vi "Parse DB - 1553 - Get BM Config.vi"(0 "channel config handle":u32, 11 "error in (no error)":errorcluster) -> (4 "channel config handle out":u32, 6 "Bus_Monitor":T1, 8 "Address Set Inverted":bool, 15 "error out":errorcluster)   [LabVIEW 2013]
uses:
  Controls/1553_Bus_Monitor.ctl
  Controls/1553_BM_Message.ctl
  Controls/664 -Param.ctl
  Controls/1553_Bus_Controller.ctl
  Controls/1553_BC_Message.ctl
  Controls/1553_Acyclic_Frame.ctl
  AIT 664 Custom Device.lvlib
  <userlib>/MIL-STD-1553/Owl1553.lvlib
panel:
  out "BM Tx Array":bool[][](array[boolean])
  out "BM Rx Array":bool[][](array[boolean])
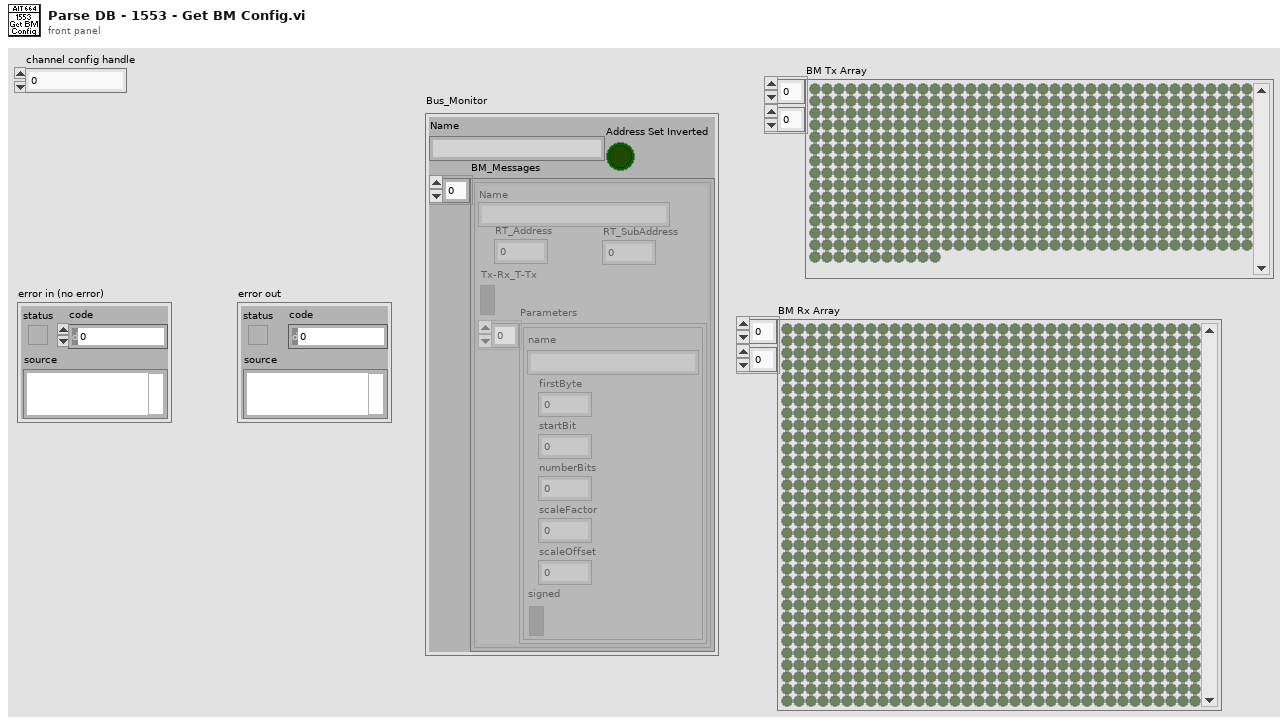
[diagram p1: front panel]
types:
  T1 = typedef "AIT 664 Custom Device.lvlib/1553_Bus_Monitor.ctl" = cluster{"Name":string, "BM_Messages":T2[], "Address Set Inverted":bool}
  T2 = typedef "AIT 664 Custom Device.lvlib/1553_BM_Message.ctl" = cluster{"RT_Address":u8, "RT_SubAddress":u8, "Tx-Rx_T-Tx":bool, "Parameters":T3[], "Name":string}
  T3 = typedef "AIT 664 Custom Device.lvlib/664 -Param.ctl" = cluster{"name":string, "firstByte":i32, "startBit":i32, "numberBits":i32, "scaleFactor":dbl, "scaleOffset":dbl, "signed":bool}
  T4 = typedef "AIT 664 Custom Device.lvlib/1553_Bus_Controller.ctl" = cluster{"BC_Messages":T5[], "Acyclic_Frames":T6[], "Enabled":bool}
  T5 = typedef "AIT 664 Custom Device.lvlib/1553_BC_Message.ctl" = cluster{"Name":string, "Tx-Rx_T-Tx":bool, "RT_Address":u8, "RT_SA_Address":u8, "Parameters":T3[], "Transfer Enabled":bool, "Message Buffer ID":u16, "Default_Message_Buffer_Data":u16[], "Word_Count":u8}
  T6 = typedef "AIT 664 Custom Device.lvlib/1553_Acyclic_Frame.ctl" = cluster{"Frame_Index":u8, "Initiate_Xfer":bool}
  T7 = enum16{"OWL1553_RECEIVE_TRANSFER", "OWL1553_TRANSMIT_TRANSFER"}
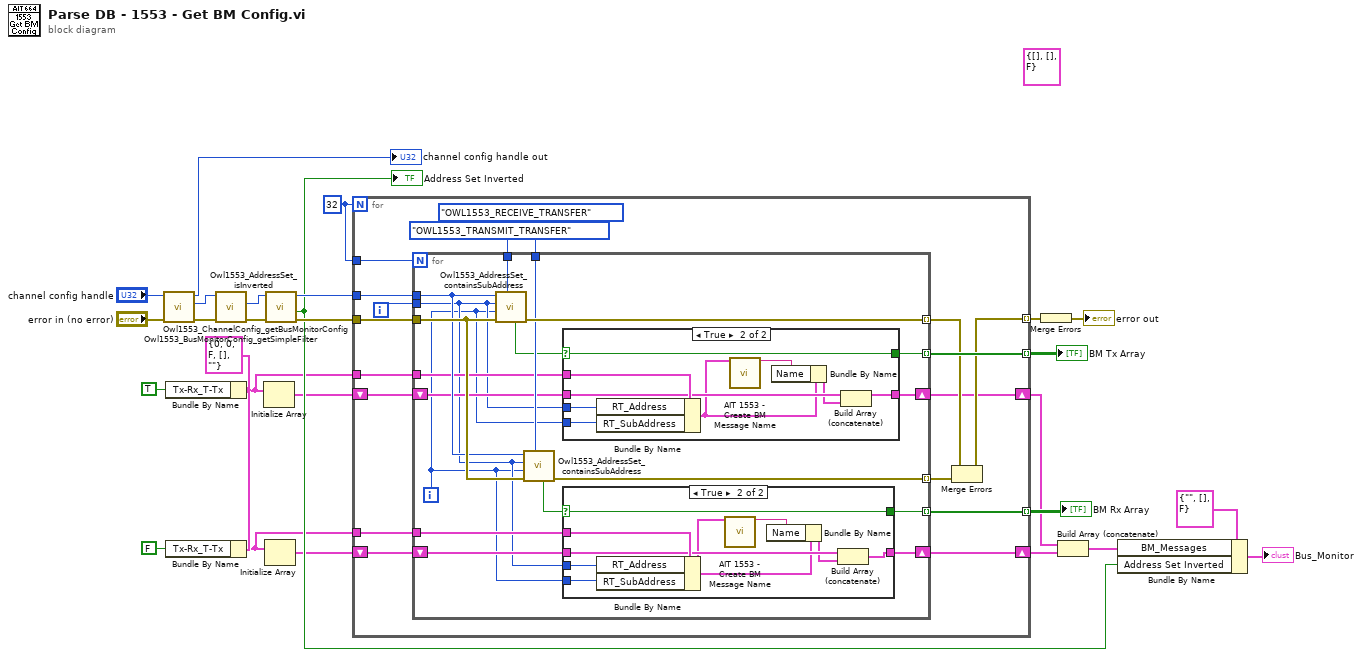
[diagram p0: block diagram]
diagram:
  w11 = T2 {"RT_Address"=0, "RT_SubAddress"=0, "Tx-Rx_T-Tx"=FALSE, "Parameters"=[], "Name"=""} ("BM_Message")
  w26 = 32
  (unwired) T4 {"BC_Messages"=[], "Acyclic_Frames"=[], "Enabled"=FALSE} ("Bus_Controller")
  n1 = call <userlib>:"Owl1553_ChannelConfig_getBusMonitorConfig.vi"("error in (no error)"="error in (no error)", "channel config handle"="channel config handle") -> ("error out"=w23:errorcluster, "bus monitor config handle"=w22:u64, "channel config handle"=→"channel config handle out":u64)  [unwired: 7 in]
  n2 = Bundle By Name(cluster=w11, "Tx-Rx_T-Tx"=TRUE ("Tx-Rx (T=Tx)")) -> (w9:T2)
  n3 = Bundle By Name(cluster=w11, "Tx-Rx_T-Tx"=FALSE ("Tx-Rx (T=Tx)")) -> (w8:T2)
  n4 = call <userlib>:"Owl1553_BusMonitorConfig_getSimpleFilter.vi"("error in (no error)"=w23, "config handle"=w22) -> ("error out"=w18:errorcluster, "address set handle"=w1:u64)  [unwired: 7 in, 1 out]
  n5 = Initialize Array(w9) -> (w14:T2[])  [unwired: 1 in]
  n6 = Initialize Array(w8) -> (w10:T2[])  [unwired: 1 in]
  n7 = call <userlib>:"Owl1553_AddressSet_isInverted.vi"("error in (no error)"=w18, "address set handle"=w1) -> ("error out"=w16:errorcluster, "inverted"=w15:bool, "address set handle"=w17:u64)  [unwired: 7 in]
  "Address Set Inverted" <- w15
  n8 = for {
    N: w26 -> [_]
    tunnel: w17 -> [w44]
    tunnel: w16 -> [w43]
    tunnel: [w34] -> w3 mode=indexing
    tunnel: [w42] -> w24 mode=indexing
    tunnel: w26 -> [w40]
    tunnel: [w37] -> w25 mode=indexing
    shift-right: [w31] -> w6
    shift-left: w14 -> [w32]
    shift-right: [w28] -> w7
    shift-left: w10 -> [w30]
    tunnel: w9 -> [w33]
    tunnel: w8 -> [w29]
    i -> [w41]
    n9 = for {
      N: w40 -> [_]
      tunnel: w44 -> [w59]
      tunnel: w43 -> [w60]
      tunnel: [w53] -> w42 mode=indexing
      tunnel: [w62] -> w35 mode=indexing
      tunnel: w41 -> [w46]
      tunnel: [w61] -> w36 mode=indexing
      tunnel: T7."OWL1553_TRANSMIT_TRANSFER" ("direction") -> [w57]
      tunnel: T7."OWL1553_RECEIVE_TRANSFER" ("direction") -> [w58]
      tunnel: [w50] -> w37 mode=indexing
      tunnel: w33 -> [w56]
      shift-right: [w52] -> w31
      shift-left: w32 -> [w55]
      shift-right: [w47] -> w28
      shift-left: w30 -> [w49]
      tunnel: w29 -> [w48]
      i -> [w45]
      n10 = call <userlib>:"Owl1553_AddressSet_containsSubAddress.vi"("direction"=w57, "error in (no error)"=w60, "sub address"=w45, "remote terminal address"=w46, "address set handle"=w59) -> ("error out"=w62:errorcluster, "contains sub-address"=w54:bool)  [unwired: 4 in, 1 out]
      n11 = call <userlib>:"Owl1553_AddressSet_containsSubAddress.vi"("direction"=w58, "error in (no error)"=w60, "sub address"=w45, "remote terminal address"=w46, "address set handle"=w59) -> ("error out"=w61:errorcluster, "contains sub-address"=w51:bool)  [unwired: 4 in, 1 out]
      n12 = case shown="True" w54 {
        selector: w54 -> [w74 w83]
        tunnel: w56 -> [_ w84]
        tunnel: w55 -> [w75 w82]
        tunnel: [w74 w83] -> w53
        tunnel: [w75 w81] -> w52
        tunnel: w46 -> [_ w80]
        tunnel: w45 -> [_ w79]
        frame False {
        }
        frame True {
          n13 = Bundle By Name(cluster=w84, "RT_Address"=w80, "RT_SubAddress"=w79) -> (w77:T2)
          n14 = call "AIT 1553 - Create BM Message Name.vi"("BM_Message"=w77) -> ("Message Name"=w78:string)  [unwired: 13 in, 1 out]
          n15 = Bundle By Name(cluster=w77, "Name"=w78) -> (w76:T2)
          n16 = Build Array (concatenate)(w82, w76) -> (w81:T2[])
        }
      }
      n17 = case shown="True" w51 {
        selector: w51 -> [w63 w72]
        tunnel: w48 -> [_ w73]
        tunnel: w49 -> [w64 w71]
        tunnel: [w63 w72] -> w50
        tunnel: [w64 w70] -> w47
        tunnel: w46 -> [_ w69]
        tunnel: w45 -> [_ w68]
        frame False {
        }
        frame True {
          n18 = Bundle By Name(cluster=w73, "RT_Address"=w69, "RT_SubAddress"=w68) -> (w66:T2)
          n19 = call "AIT 1553 - Create BM Message Name.vi"("BM_Message"=w66) -> ("Message Name"=w67:string)  [unwired: 13 in, 1 out]
          n20 = Bundle By Name(cluster=w66, "Name"=w67) -> (w65:T2)
          n21 = Build Array (concatenate)(w71, w65) -> (w70:T2[])
        }
      }
    }
    n22 = Merge Errors(w35, w36) -> (w34:errorcluster)
  }
  "BM Tx Array" <- w24
  "BM Rx Array" <- w25
  n23 = Merge Errors(w3) -> (→"error out":errorcluster)
  n24 = Build Array (concatenate)(w6, w7) -> (w5:T2[])
  n25 = Bundle By Name(cluster=T1 {"Name"="", "BM_Messages"=[], "Address Set Inverted"=FALSE} ("Bus_Monitor"), "BM_Messages"=w5, "Address Set Inverted"=w15) -> (→"Bus_Monitor":T1)
